vi "test_Multiple Periodic Command Message.vi"(8 "error in (no error)":errorcluster, 11 "TestCase in":refnum<class "Instrument Addon Common System Tests.lvclass">) -> (0 "error out":errorcluster, 3 "TestCase out":refnum<class "Instrument Addon Common System Tests.lvclass">)   [LabVIEW 2018, in "Instrument Addon Common System Tests.lvclass"]
uses:
  Instrument Addon Common System Tests.lvclass
  C:/Users/nitest/Git/NI VS Test Utilities/VeriStandTestCase/VeriStandTestCase.lvclass
  4b26bf46-6d54-4276-a8e8-45773f49de4b.vi
  <vilib>/addons/_JKI Toolkits/VI Tester/TestCase.llb/TestCase.lvclass
  C:/Program Files (x86)/National Instruments/LabVIEW 2018/vi.lib/addons/_JKI Toolkits/VI Tester/TestCase.llb/TestCase.lvclass
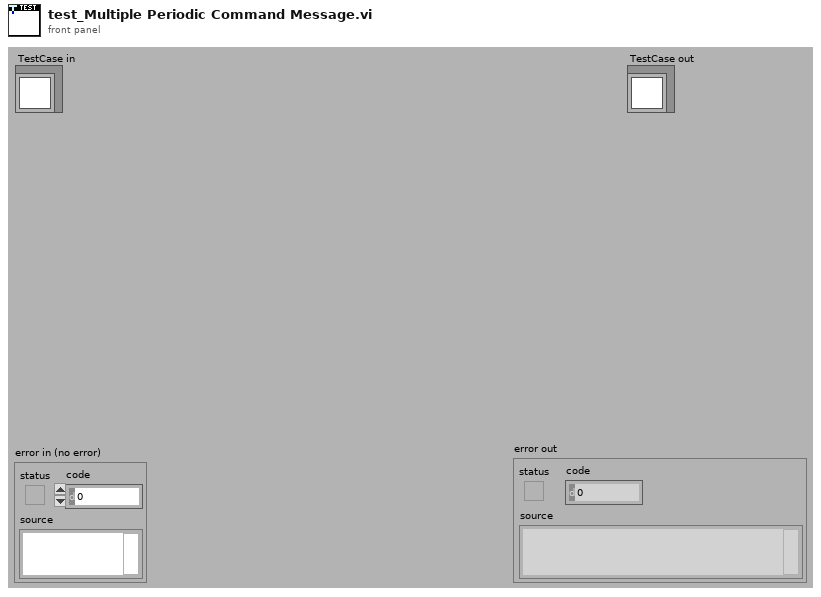
[diagram p1: front panel]
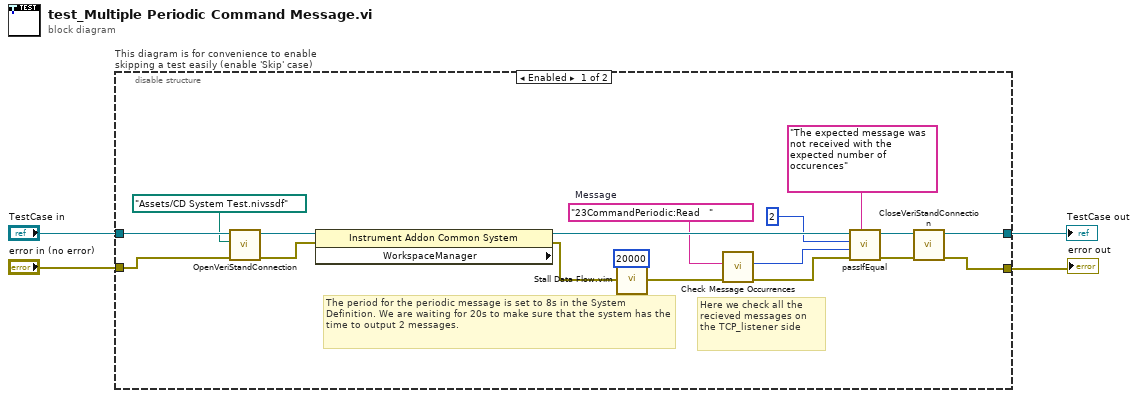
[diagram p0: block diagram]
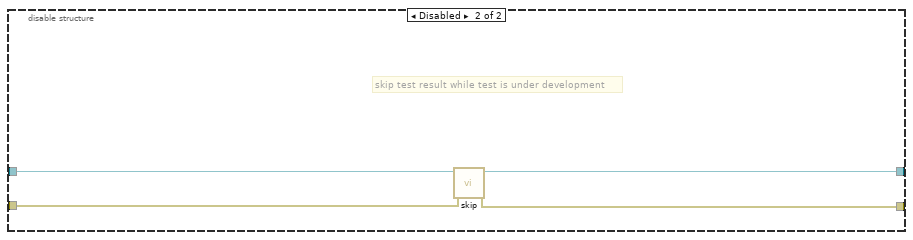
[diagram p2: hidden frame]
diagram:
  n1 = disable-structure "This diagram is for convenience to enable skipping a test easily (enable 'Skip' case)" shown="Enabled" {
    disable-tunnel: "TestCase in" -> [w20 w26]
    disable-tunnel: [w21 w24] -> w2
    disable-tunnel: [w22 w25] -> w1
    disable-tunnel: "error in (no error)" -> [w18 w23]
    frame Enabled {
      w8 = "23CommandPeriodic:Read   "  # Message
      # "The period for the periodic message is set to 8s in the System Definition. We are waiting for 20s to make sure that the system has the time to output 2 messages."
      # "Here we check all the recieved messages on the TCP_listener side"
      n2 = call-dynamic "OpenVeriStandConnection.vi"("error in (no error)"=w18, "System Definition File"=path "Assets/CD System Test.nivssdf", "VeriStand Test Case in"=w20) -> ("error out"=w17:errorcluster, "VeriStand Test Case out"=w19:refnum<class "Instrument Addon Common System Tests.lvclass">)  [unwired: 6 in, 1 out]
      n3 = property class="Instrument Addon Common System " props=["WorkspaceManager"](reference=w19, error in=w17) -> (reference out=w14:refnum<class "Instrument Addon Common System Tests.lvclass">, error out=w7:errorcluster)  [unwired: 1 out]
      n4 = call "Stall Data Flow.vim"("value in"=w7, "milliseconds to wait"=u32 20000) -> ("value out"=w6:errorcluster)  [unwired: 1 out]
      n5 = call "Check Message Occurrences.vi"("error in (no error)"=w6, "Message"=w8) -> ("error IO"=w15:errorcluster, "Occurences"=w10:i32)  [unwired: 8 in]
      n6 = call-dynamic "passIfEqual.vi"("custom report message (\"\")"="The expected message was not received with the expected number of occurences" ("custom report message (\"\")"), "error in (no error)"=w15, "y"=w10, "x"=2, "TestCase in"=w14) -> ("error out"=w12:errorcluster, "TestCase out"=w13:refnum<class "Instrument Addon Common System Tests.lvclass">)  [unwired: 5 in]
      n7 = call-dynamic "CloseVeriStandConnection.vi"("error in (no error)"=w12, "VeriStand Test Case in"=w13) -> ("error out"=w22:errorcluster, "VeriStand Test Case out"=w21:refnum<class "Instrument Addon Common System Tests.lvclass">)  [unwired: 8 in]
    }
    frame Disabled {
      # "skip test result while test is under development"
      n8 = call <vilib>:"skip.vi"("error in (no error)"=w23, "TestCase in"=w26) -> ("error out"=w25:errorcluster, "TestCase out"=w24:refnum<class "Instrument Addon Common System Tests.lvclass">)  [unwired: 8 in]
    }
  }
  "error out" <- w1
  "TestCase out" <- w2
